vi "writeYearMonth.vi"(8 "error in (no error)":errorcluster, 9 "Month":i32, 10 "Year":i32, 11 "MonthDisplay in":refnum<class "DateUserInterface.lvclass">) -> (0 "error out":errorcluster, 3 "MonthDisplay out":refnum<class "DateUserInterface.lvclass">)   [LabVIEW 2018, in "DateUserInterface.lvclass"]
uses:
  DateUserInterface.lvclass
  month.ctl
  DateUserInterface.lvclass/DateUserInterface.ctl
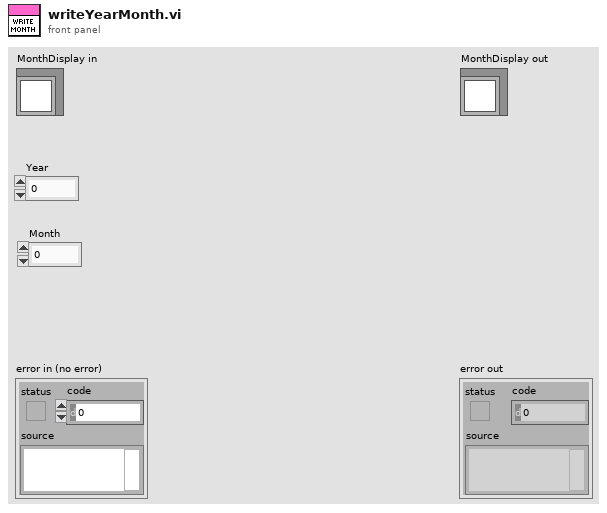
[diagram p1: front panel]
types:
  T1 = typedef "DateUserInterface.lvclass/month.ctl" = enum16{"January", "February", "March", "April", "May", "June", "July", "August", "September", "October", "November", "December"}
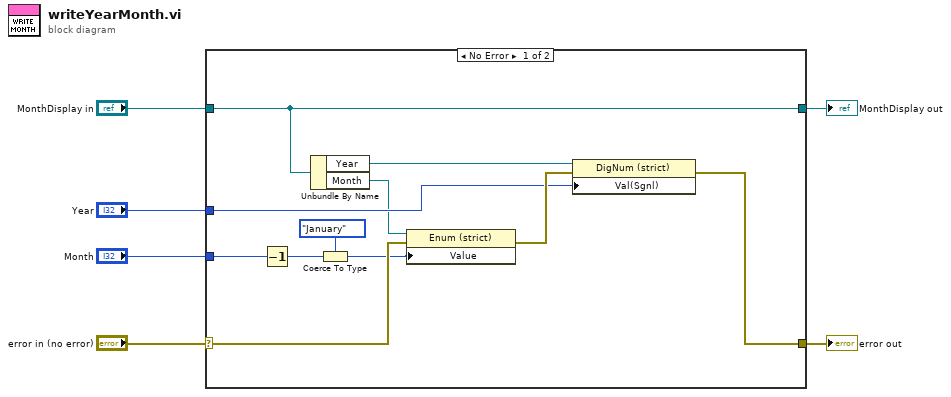
[diagram p0: block diagram]
diagram:
  n1 = case shown="No Error" "error in (no error)" {
    selector: "error in (no error)" -> [w15 w19]
    tunnel: [w11 w19] -> w5
    tunnel: [w17 w18] -> w3
    tunnel: "MonthDisplay in" -> [w17 w18]
    tunnel: "Month" -> [w13 _]
    tunnel: "Year" -> [w12 _]
    frame No Error {
      n2 = Decrement(x=w13) -> (x-1=w10:i32)
      n3 = Unbundle By Name(w17) -> ("Year"=w16:refnum<vi>, "Month"=w7:refnum<vi>)
      n4 = Coerce To Type(0:w10, 1:month."January" ("Month")) -> (2:w8:T1)
      n5 = property class="Enum (strict)"(reference=w7, error in=w15, "Value"=w8) -> (error out=w14:errorcluster)  [unwired: 1 out]
      n6 = property class="DigNum (strict)"(reference=w16, error in=w14, "Val(Sgnl)"=w12) -> (error out=w11:errorcluster)  [unwired: 1 out]
    }
    frame Error {
    }
  }
  "error out" <- w5
  "MonthDisplay out" <- w3
